vi "Galvo Parameters - FGV.vi"(7 "Actions":T19=enum."Clear", 8 "Error In":errorcluster, 10 "Galvo parameters in":T1={"System Parameters"={"Optical Parameters"={"Obj. Focal Length [mm]"=45.0, "Scan Lens EFL[mm]"=59.5, "Tube Lens EFL[mm]"=205.0, "Galvo V Range (+/-)"=10.0, "Galvo Max Half Angle [Deg]"=19.0, "Max Galvo Range[%]"=0.0}, "Vibratome"={"Z Bottom [mm]"=0.0, "Pre Cut Dwell [s]"=0.0, "Blade Frequency [RPM]"=0, "Slice Speed [mm/s]"=0.0, "Post Cut Dwell [s]"=0.0, "Ramp Time [s]"=0.0, "Start X [mm]"=0.0, "Start Y [mm]"=0.0, "Slice Length [mm]"=0.0, "Slice Axis"=enum."Y Axis", "Controller VISA Ref"="COM4"}, "Table Stages"={"X Stage"={"Position"=0.0, "Is.Enabled?"=FALSE, "Is.Connected?"=FALSE, "Device SN"="45876539", "AccelerationMaximum"=0.0, "VelocityMaximum"=0.0, "Acceleration"=0.0, "Velocity"=0.0, "waitTimeout (ms)"=0, "Model"=enum."None", "Is.Homed?"=FALSE}, "Y Stage"={"Position"=0.0, "Is.Enabled?"=FALSE, "Is.Connected?"=FALSE, "Device SN"="45876539", "AccelerationMaximum"=0.0, "VelocityMaximum"=0.0, "Acceleration"=0.0, "Velocity"=0.0, "waitTimeout (ms)"=0, "Model"=enum."None", "Is.Homed?"=FALSE}, "Z Stage"={"Position"=0.0, "Is.Enabled?"=FALSE, "Is.Connected?"=FALSE, "Device SN"="45876539", "AccelerationMaximum"=0.0, "VelocityMaximum"=0.0, "Acceleration"=0.0, "Velocity"=0.0, "waitTimeout (ms)"=0, "Model"=enum."None", "Is.Homed?"=FALSE}}, "Imaging Parameter"={"Raster Scan Direction"=enum."Uni Directional", "Pixel Dwell Time [Clock Cycles]"=1, "Flyback Time [Clock Cycles]"=200, "XY Center [um]"={"X"=1.0, "Y"=1.0}, "Pixel Step Size [um]"=2.5, "XY Image Size"=enum."2048 x 2048", "Custom"=FALSE, "Custom Size"={"X"=10, "Y"=10}, "Line Averages"=1}, "Galvo HW Parameters"={"Analog Out Channel"="GalvoCtrl/ao0,GalvoCtrl/ao1", "Min Voltage"=-10.0, "Max Voltage"=10.0, "Pixel Clock Source"="/GalvoCtrl/PFI0", "Sample Rate"=1000.0, "Line Clock Out Ch"="GalvoCtrl/port0/line0"}, "Alazar parameters"={"Trigger Settings"={"General Trigger Settings"={"Trigger Operation"=0, "Coupling ID"=2, "Range ID"=2, "Delay"=0, "Timeout Ticks"=0, "Mode"=1, "Parameter"=1}, "Trigger Engine 1"={"Trigger Engine"=0, "Source"=2, "Slope"=1, "Level"=140}, "Trigger Engine 2"={"Trigger Engine"=1, "Source"=3, "Slope"=1, "Level"=140}}, "Capture Clock"={"Sample Rate"=100, "Decimation"=0, "Source"=2, "Edge"=0}, "Device ID"={"System ID"=1, "Board ID"=1}, "Ch A Input Control"={"Channel"=1, "Coupling"=2, "Range"=10, "Impedance"=2}, "Ch B Input Control"={"Channel"=2, "Coupling"=2, "Range"=10, "Impedance"=2}, "Acq Settings"={"Window Type"=1, "Record Length"=1440, "Footer"=0, "Output Format"=10, "Offset"=0, "Records Per Buffer"=2048, "Samples per record"=2048, "Records Count (Records/Acq)"=2147483647}, "Cluster"={"FFT value magnification"=1000.0, "max queue size (-1, unlimited)"=-1, "File Type"=enum."Tiff", "file path"=path "C:/Users/BoasLab/Documents/Data/Alazar data/B-line/data/test.tif", "#A-lines to save"=2048, "#Z pixels to save"=2048, "ImageDescription"="", "Convert to U16?"=FALSE}}}} {"System Parameters"."Alazar parameters"."Cluster"."FFT value magnification" min=0.0 max=10000.0 step=0.001 format="%.4f"; "System Parameters"."Alazar parameters"."Acq Settings"."Window Type" items=["DSP_WINDOW_NONE", "DSP_WINDOW_HANNING", "DSP_WINDOW_HAMMING", "DSP_WINDOW_BLACKMAN", "DSP_WINDOW_BLACKMAN_HARRIS", "DSP_WINDOW_BARTLETT"]; "System Parameters"."Alazar parameters"."Acq Settings"."Footer" items=["FOOTER_NONE", "FOOTER_NPT"]; "System Parameters"."Alazar parameters"."Acq Settings"."Output Format" items=["FLOAT_AMP2"=10, "FLOAT_LOG"=11]; "System Parameters"."Alazar parameters"."Ch B Input Control"."Channel" items=["A"=1, "B"=2, "C"=4, "D"=8]; "System Parameters"."Alazar parameters"."Ch B Input Control"."Coupling" items=["AC"=1, "DC"=2]; "System Parameters"."Alazar parameters"."Ch B Input Control"."Range" items=["20 mV"=1, "40 mV"=2, "50 mV"=3, "80 mV"=4, "100 mV"=5, "200 mV"=6, "400 mV"=7, "500 mV"=8, "800 mV"=9, "1 V"=10, "1.25 V"=33, "2 V"=11, "4 V"=12, "5 V"=13, "8 V"=14, "10 V"=15, "20 V"=16]; "System Parameters"."Alazar parameters"."Ch B Input Control"."Impedance" items=["1 MOhm"=1, "50 Ohm"=2, ""=0]; "System Parameters"."Alazar parameters"."Ch A Input Control"."Channel" items=["A"=1, "B"=2, "C"=4, "D"=8]; "System Parameters"."Alazar parameters"."Ch A Input Control"."Coupling" items=["AC"=1, "DC"=2]; "System Parameters"."Alazar parameters"."Ch A Input Control"."Range" items=["20 mV"=1, "40 mV"=2, "50 mV"=3, "80 mV"=4, "100 mV"=5, "200 mV"=6, "400 mV"=7, "500 mV"=8, "800 mV"=9, "1 V"=10, "1.25 V"=33, "2 V"=11, "4 V"=12, "5 V"=13, "8 V"=14, "10 V"=15, "20 V"=16]; "System Parameters"."Alazar parameters"."Ch A Input Control"."Impedance" items=["1 MOhm"=1, "50 Ohm"=2, ""=0]; "System Parameters"."Alazar parameters"."Capture Clock"."Edge" items=["Rising", "Falling"]; "System Parameters"."Alazar parameters"."Capture Clock"."Source" items=["Internal"=1, "Fast External"=2, "Medium External"=3, "Slow External"=4, "External AC"=5, "External DC"=6, "External 10MHz"=7]; "System Parameters"."Alazar parameters"."Trigger Settings"."General Trigger Settings"."Trigger Operation" items=["J", "K", "J OR K", "J AND K", "J XOR K", "J AND NOT K", "NOT J AND K"]; "System Parameters"."Alazar parameters"."Trigger Settings"."General Trigger Settings"."Coupling ID" items=["AC"=1, "DC"=2]; "System Parameters"."Alazar parameters"."Trigger Settings"."General Trigger Settings"."Range ID" items=["5 V", "1 V", "TTL"]; "System Parameters"."Alazar parameters"."Trigger Settings"."Trigger Engine 1"."Trigger Engine" items=["J", "K"]; "System Parameters"."Alazar parameters"."Trigger Settings"."Trigger Engine 1"."Source" items=["A", "B", "External", "Disable", "C", "D"]; "System Parameters"."Alazar parameters"."Trigger Settings"."Trigger Engine 1"."Slope" items=["Positive"=1, "Negative"=2]; "System Parameters"."Alazar parameters"."Trigger Settings"."Trigger Engine 2"."Trigger Engine" items=["J", "K"]; "System Parameters"."Alazar parameters"."Trigger Settings"."Trigger Engine 2"."Source" items=["A", "B", "External", "Disable", "C", "D"]; "System Parameters"."Alazar parameters"."Trigger Settings"."Trigger Engine 2"."Slope" items=["Positive"=1, "Negative"=2]; "System Parameters"."Imaging Parameter"."Line Averages" min=1 max=30 step=1; "System Parameters"."Imaging Parameter"."Flyback Time [Clock Cycles]" max=10 step=1; "System Parameters"."Imaging Parameter"."Pixel Step Size [um]" min=0.0 max=10.0 step=0.01; "System Parameters"."Imaging Parameter"."Custom Size"."Y" min=1 max=30 step=1; "System Parameters"."Imaging Parameter"."Custom Size"."X" min=1 max=30 step=1; "System Parameters"."Imaging Parameter"."XY Center [um]"."Y" min=1.0 max=30.0 step=1.0; "System Parameters"."Imaging Parameter"."XY Center [um]"."X" min=1.0 max=30.0 step=1.0; "System Parameters"."Imaging Parameter"."Pixel Dwell Time [Clock Cycles]" max=10 step=1}) -> (0 "Error Out":errorcluster, 2 "Galvo parameters out":T1={"System Parameters"={"Optical Parameters"={"Obj. Focal Length [mm]"=45.0, "Scan Lens EFL[mm]"=59.5, "Tube Lens EFL[mm]"=205.0, "Galvo V Range (+/-)"=10.0, "Galvo Max Half Angle [Deg]"=19.0, "Max Galvo Range[%]"=0.0}, "Vibratome"={"Z Bottom [mm]"=0.0, "Pre Cut Dwell [s]"=0.0, "Blade Frequency [RPM]"=0, "Slice Speed [mm/s]"=0.0, "Post Cut Dwell [s]"=0.0, "Ramp Time [s]"=0.0, "Start X [mm]"=0.0, "Start Y [mm]"=0.0, "Slice Length [mm]"=0.0, "Slice Axis"=enum."Y Axis", "Controller VISA Ref"="COM4"}, "Table Stages"={"X Stage"={"Position"=0.0, "Is.Enabled?"=FALSE, "Is.Connected?"=FALSE, "Device SN"="45876539", "AccelerationMaximum"=0.0, "VelocityMaximum"=0.0, "Acceleration"=0.0, "Velocity"=0.0, "waitTimeout (ms)"=0, "Model"=enum."None", "Is.Homed?"=FALSE}, "Y Stage"={"Position"=0.0, "Is.Enabled?"=FALSE, "Is.Connected?"=FALSE, "Device SN"="45876539", "AccelerationMaximum"=0.0, "VelocityMaximum"=0.0, "Acceleration"=0.0, "Velocity"=0.0, "waitTimeout (ms)"=0, "Model"=enum."None", "Is.Homed?"=FALSE}, "Z Stage"={"Position"=0.0, "Is.Enabled?"=FALSE, "Is.Connected?"=FALSE, "Device SN"="45876539", "AccelerationMaximum"=0.0, "VelocityMaximum"=0.0, "Acceleration"=0.0, "Velocity"=0.0, "waitTimeout (ms)"=0, "Model"=enum."None", "Is.Homed?"=FALSE}}, "Imaging Parameter"={"Raster Scan Direction"=enum."Uni Directional", "Pixel Dwell Time [Clock Cycles]"=1, "Flyback Time [Clock Cycles]"=200, "XY Center [um]"={"X"=1.0, "Y"=1.0}, "Pixel Step Size [um]"=2.5, "XY Image Size"=enum."2048 x 2048", "Custom"=FALSE, "Custom Size"={"X"=10, "Y"=10}, "Line Averages"=1}, "Galvo HW Parameters"={"Analog Out Channel"="GalvoCtrl/ao0,GalvoCtrl/ao1", "Min Voltage"=-10.0, "Max Voltage"=10.0, "Pixel Clock Source"="/GalvoCtrl/PFI0", "Sample Rate"=1000.0, "Line Clock Out Ch"="GalvoCtrl/port0/line0"}, "Alazar parameters"={"Trigger Settings"={"General Trigger Settings"={"Trigger Operation"=0, "Coupling ID"=2, "Range ID"=2, "Delay"=0, "Timeout Ticks"=0, "Mode"=1, "Parameter"=1}, "Trigger Engine 1"={"Trigger Engine"=0, "Source"=2, "Slope"=1, "Level"=140}, "Trigger Engine 2"={"Trigger Engine"=1, "Source"=3, "Slope"=1, "Level"=140}}, "Capture Clock"={"Sample Rate"=100, "Decimation"=0, "Source"=2, "Edge"=0}, "Device ID"={"System ID"=1, "Board ID"=1}, "Ch A Input Control"={"Channel"=1, "Coupling"=2, "Range"=10, "Impedance"=2}, "Ch B Input Control"={"Channel"=2, "Coupling"=2, "Range"=10, "Impedance"=2}, "Acq Settings"={"Window Type"=1, "Record Length"=1440, "Footer"=0, "Output Format"=10, "Offset"=0, "Records Per Buffer"=2048, "Samples per record"=2048, "Records Count (Records/Acq)"=2147483647}, "Cluster"={"FFT value magnification"=1000.0, "max queue size (-1, unlimited)"=-1, "File Type"=enum."Tiff", "file path"=path "C:/Users/BoasLab/Documents/Data/Alazar data/B-line/data/test.tif", "#A-lines to save"=2048, "#Z pixels to save"=2048, "ImageDescription"="", "Convert to U16?"=FALSE}}}} {"System Parameters"."Alazar parameters"."Cluster"."FFT value magnification" min=0.0 max=10000.0 step=0.001 format="%.4f"; "System Parameters"."Alazar parameters"."Acq Settings"."Window Type" items=["DSP_WINDOW_NONE", "DSP_WINDOW_HANNING", "DSP_WINDOW_HAMMING", "DSP_WINDOW_BLACKMAN", "DSP_WINDOW_BLACKMAN_HARRIS", "DSP_WINDOW_BARTLETT"]; "System Parameters"."Alazar parameters"."Acq Settings"."Footer" items=["FOOTER_NONE", "FOOTER_NPT"]; "System Parameters"."Alazar parameters"."Acq Settings"."Output Format" items=["FLOAT_AMP2"=10, "FLOAT_LOG"=11]; "System Parameters"."Alazar parameters"."Ch B Input Control"."Channel" items=["A"=1, "B"=2, "C"=4, "D"=8]; "System Parameters"."Alazar parameters"."Ch B Input Control"."Coupling" items=["AC"=1, "DC"=2]; "System Parameters"."Alazar parameters"."Ch B Input Control"."Range" items=["20 mV"=1, "40 mV"=2, "50 mV"=3, "80 mV"=4, "100 mV"=5, "200 mV"=6, "400 mV"=7, "500 mV"=8, "800 mV"=9, "1 V"=10, "1.25 V"=33, "2 V"=11, "4 V"=12, "5 V"=13, "8 V"=14, "10 V"=15, "20 V"=16]; "System Parameters"."Alazar parameters"."Ch B Input Control"."Impedance" items=["1 MOhm"=1, "50 Ohm"=2, ""=0]; "System Parameters"."Alazar parameters"."Ch A Input Control"."Channel" items=["A"=1, "B"=2, "C"=4, "D"=8]; "System Parameters"."Alazar parameters"."Ch A Input Control"."Coupling" items=["AC"=1, "DC"=2]; "System Parameters"."Alazar parameters"."Ch A Input Control"."Range" items=["20 mV"=1, "40 mV"=2, "50 mV"=3, "80 mV"=4, "100 mV"=5, "200 mV"=6, "400 mV"=7, "500 mV"=8, "800 mV"=9, "1 V"=10, "1.25 V"=33, "2 V"=11, "4 V"=12, "5 V"=13, "8 V"=14, "10 V"=15, "20 V"=16]; "System Parameters"."Alazar parameters"."Ch A Input Control"."Impedance" items=["1 MOhm"=1, "50 Ohm"=2, ""=0]; "System Parameters"."Alazar parameters"."Capture Clock"."Edge" items=["Rising", "Falling"]; "System Parameters"."Alazar parameters"."Capture Clock"."Source" items=["Internal"=1, "Fast External"=2, "Medium External"=3, "Slow External"=4, "External AC"=5, "External DC"=6, "External 10MHz"=7]; "System Parameters"."Alazar parameters"."Trigger Settings"."General Trigger Settings"."Trigger Operation" items=["J", "K", "J OR K", "J AND K", "J XOR K", "J AND NOT K", "NOT J AND K"]; "System Parameters"."Alazar parameters"."Trigger Settings"."General Trigger Settings"."Coupling ID" items=["AC"=1, "DC"=2]; "System Parameters"."Alazar parameters"."Trigger Settings"."General Trigger Settings"."Range ID" items=["5 V", "1 V", "TTL"]; "System Parameters"."Alazar parameters"."Trigger Settings"."Trigger Engine 1"."Trigger Engine" items=["J", "K"]; "System Parameters"."Alazar parameters"."Trigger Settings"."Trigger Engine 1"."Source" items=["A", "B", "External", "Disable", "C", "D"]; "System Parameters"."Alazar parameters"."Trigger Settings"."Trigger Engine 1"."Slope" items=["Positive"=1, "Negative"=2]; "System Parameters"."Alazar parameters"."Trigger Settings"."Trigger Engine 2"."Trigger Engine" items=["J", "K"]; "System Parameters"."Alazar parameters"."Trigger Settings"."Trigger Engine 2"."Source" items=["A", "B", "External", "Disable", "C", "D"]; "System Parameters"."Alazar parameters"."Trigger Settings"."Trigger Engine 2"."Slope" items=["Positive"=1, "Negative"=2]; "System Parameters"."Imaging Parameter"."Line Averages" min=1 max=30 step=1; "System Parameters"."Imaging Parameter"."Flyback Time [Clock Cycles]" max=10 step=1; "System Parameters"."Imaging Parameter"."Pixel Step Size [um]" min=0.0 max=10.0 step=0.01; "System Parameters"."Imaging Parameter"."Custom Size"."Y" min=1 max=30 step=1; "System Parameters"."Imaging Parameter"."Custom Size"."X" min=1 max=30 step=1; "System Parameters"."Imaging Parameter"."XY Center [um]"."Y" min=1.0 max=30.0 step=1.0; "System Parameters"."Imaging Parameter"."XY Center [um]"."X" min=1.0 max=30.0 step=1.0; "System Parameters"."Imaging Parameter"."Pixel Dwell Time [Clock Cycles]" max=10 step=1})   [LabVIEW 2018]
uses:
  Controls/FGV Actions.ctl
  type defines/Galvo parameters.ctl
  Controls/System Parameters.ctl
  Controls/Optical Parameters.ctl
  Controls/Vibratome Parameters.ctl
  Controls/Translation Stage Parameters.ctl
  Hardware Mfg/Thorlabs Translation Stages/Controls/Translation Stage Cluster.ctl
  Controls/Translation Stage Types.ctl
  Controls/Imaging Parameters.ctl
  Controls/Scan Direction.ctl
  type defines/Alazar parameters.ctl
  Hardware Mfg/AlazarTech SDK/Controls/General Trigger Settings.ctl
  Hardware Mfg/AlazarTech SDK/Controls/Trigger Engine Controls.ctl
  Hardware Mfg/AlazarTech SDK/Controls/Clock Controls.ctl
  Hardware Mfg/AlazarTech SDK/Controls/Alazar Device ID.ctl
  Hardware Mfg/AlazarTech SDK/Controls/Channel Input Controls.ctl
  Hardware Mfg/AlazarTech SDK/Controls/Alazar Acquisition Settings.ctl
  Controls/Control cluster.ctl
  type defines/file type.ctl
panel:
  # "X"
  # "X"
  # "X"
  # "X"
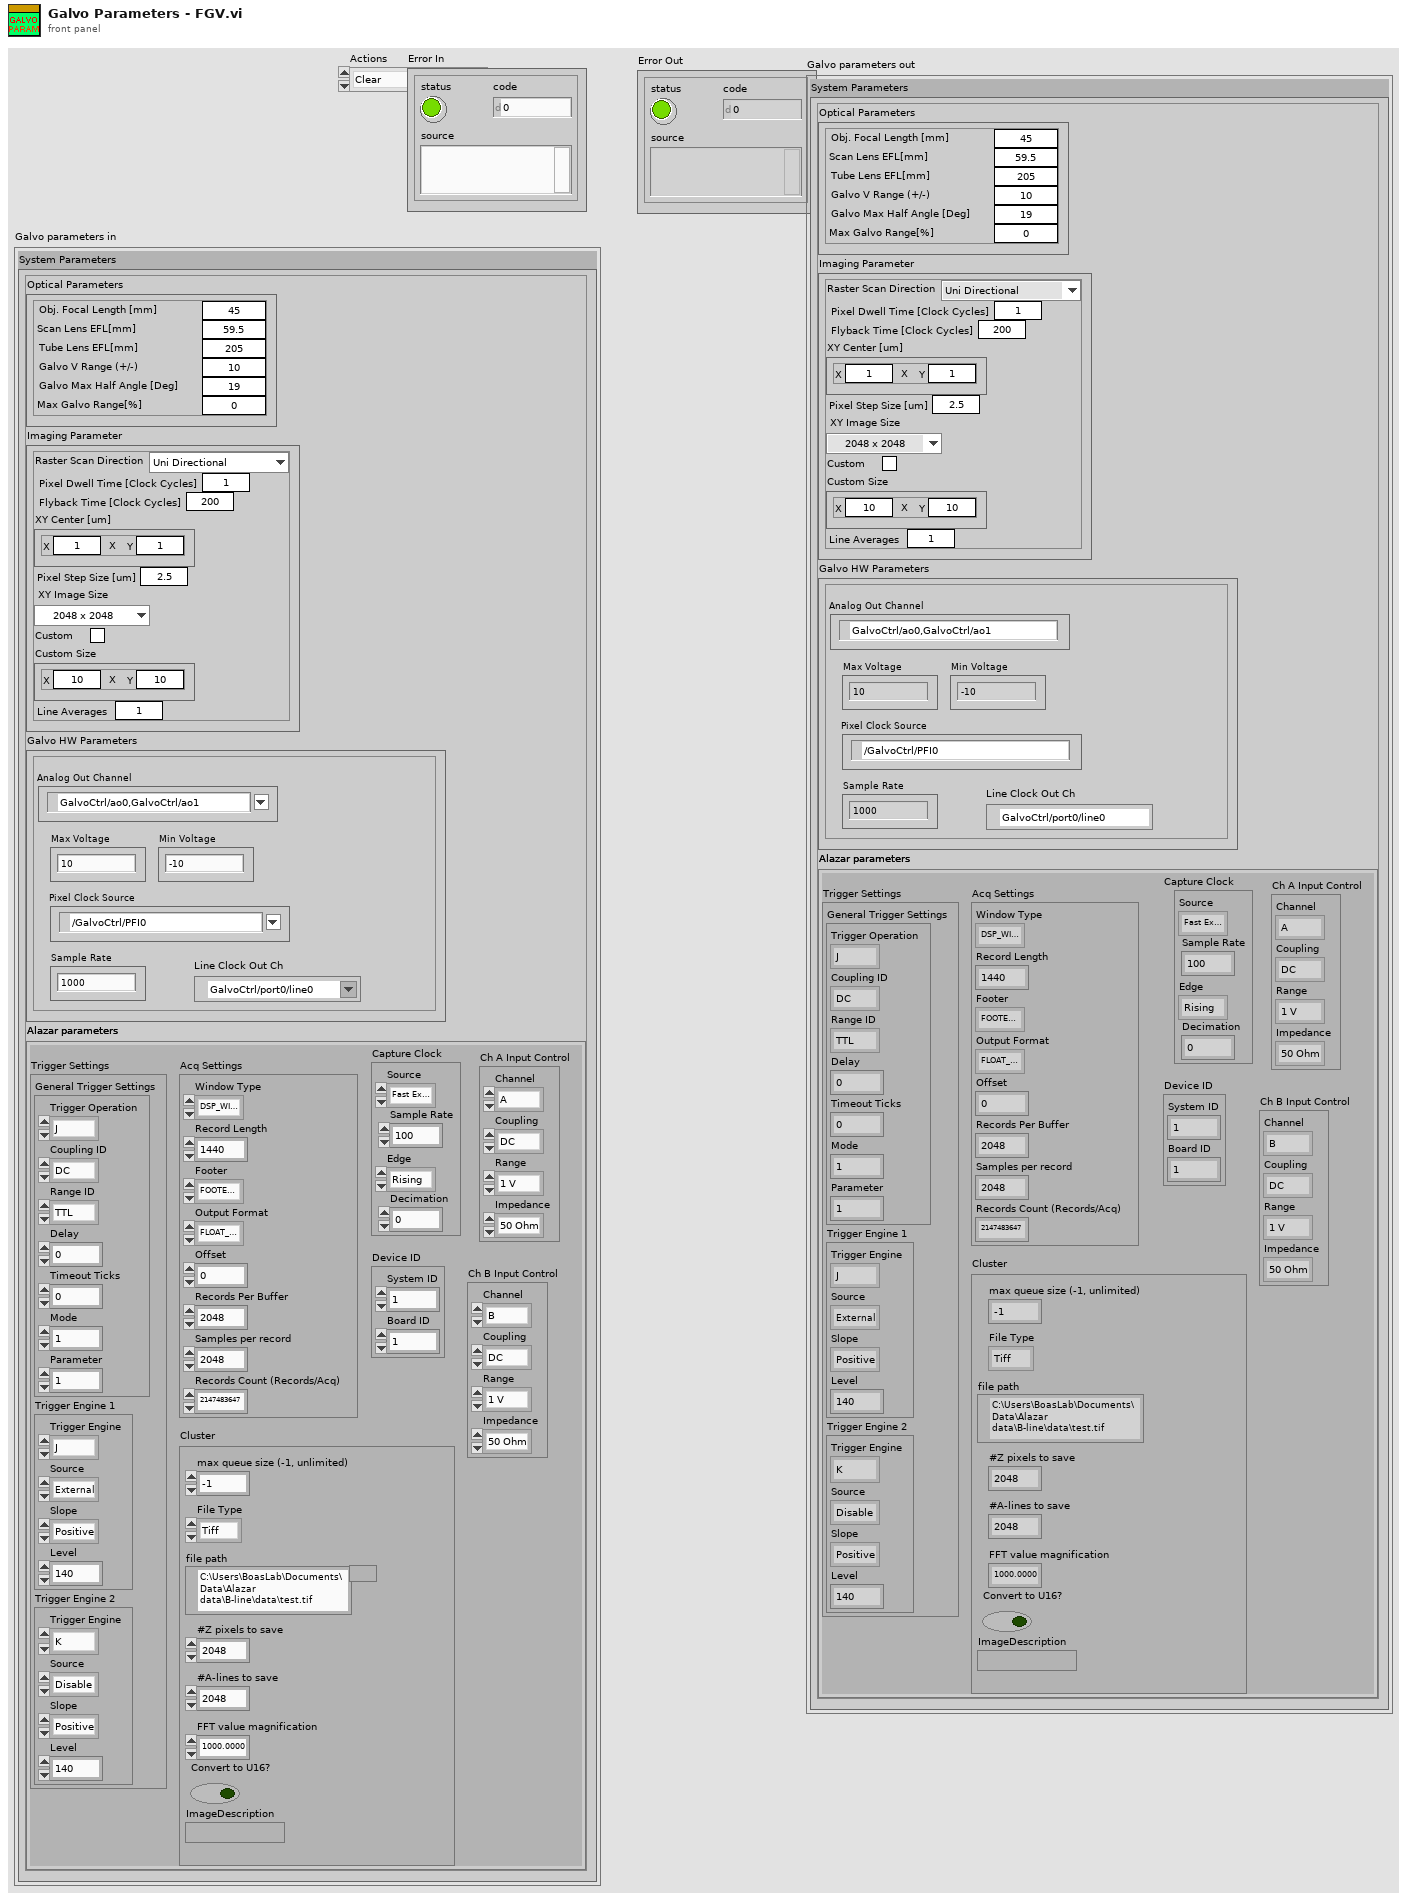
[diagram p1: front panel]
types:
  T1 = typedef "Galvo parameters.ctl" = cluster{"System Parameters":T2}
  T2 = typedef "System Parameters.ctl" = cluster{"Optical Parameters":T3, "Vibratome":T4, "Table Stages":T5, "Imaging Parameter":T8, "Galvo HW Parameters":cluster{"Analog Out Channel":tag, "Min Voltage":dbl, "Max Voltage":dbl, "Pixel Clock Source":tag, "Sample Rate":dbl, "Line Clock Out Ch":tag}, "Alazar parameters":T10}
  T3 = typedef "Optical Parameters.ctl" = cluster{"Obj. Focal Length [mm]":dbl, "Scan Lens EFL[mm]":dbl, "Tube Lens EFL[mm]":dbl, "Galvo V Range (+/-)":dbl, "Galvo Max Half Angle [Deg]":dbl, "Max Galvo Range[%]":dbl}
  T4 = typedef "Vibratome Parameters.ctl" = cluster{"Z Bottom [mm]":dbl, "Pre Cut Dwell [s]":dbl, "Blade Frequency [RPM]":u16, "Slice Speed [mm/s]":dbl, "Post Cut Dwell [s]":dbl, "Ramp Time [s]":dbl, "Start X [mm]":dbl, "Start Y [mm]":dbl, "Slice Length [mm]":dbl, "Slice Axis":enum16{"X Axis", "Y Axis", "Z Axis"}, "Controller VISA Ref":refnum<visa-resource-name>}
  T5 = typedef "Translation Stage Parameters.ctl" = cluster{"X Stage":T6, "Y Stage":T6, "Z Stage":T6}
  T6 = typedef "Translation Stage Cluster.ctl" = cluster{"Position":dbl, "Is.Enabled?":bool, "Is.Connected?":bool, "Device SN":string, "AccelerationMaximum":dbl, "VelocityMaximum":dbl, "Acceleration":dbl, "Velocity":dbl, "waitTimeout (ms)":i32, "Model":T7, "Is.Homed?":bool}
  T7 = typedef "Translation Stage Types.ctl" = enum16{"None", "Thorlabs LTS", "Thorlabs MLJ"}
  T8 = typedef "Imaging Parameters.ctl" = cluster{"Raster Scan Direction":T9, "Pixel Dwell Time [Clock Cycles]":u16, "Flyback Time [Clock Cycles]":u16, "XY Center [um]":cluster{"X":dbl, "Y":dbl}, "Pixel Step Size [um]":dbl, "XY Image Size":enum16{"32 x 32", "64 x 64", "128 x 128", "256 x 256", "512 x 512", "1024 x 1024", "2048 x 2048"}, "Custom":bool, "Custom Size":cluster{"X":u16, "Y":u16}, "Line Averages":u8}
  T9 = typedef "Scan Direction.ctl" = enum16{"Uni Directional", "Bi Directional", "None"}
  T10 = typedef "Alazar parameters.ctl" = cluster{"Trigger Settings":cluster{"General Trigger Settings":T11, "Trigger Engine 1":T12, "Trigger Engine 2":T12}, "Capture Clock":T13, "Device ID":T14, "Ch A Input Control":T15, "Ch B Input Control":T15, "Acq Settings":T16, "Cluster":T17}
  T11 = typedef "General Trigger Settings.ctl" = cluster{"Trigger Operation":u32, "Coupling ID":u32, "Range ID":u32, "Delay":u32, "Timeout Ticks":u32, "Mode":u32, "Parameter":u32}
  T12 = typedef "Trigger Engine Controls.ctl" = cluster{"Trigger Engine":u32, "Source":u32, "Slope":u32, "Level":u32}
  T13 = typedef "Clock Controls.ctl" = cluster{"Sample Rate":u32, "Decimation":u32, "Source":u32, "Edge":u32}
  T14 = typedef "Alazar Device ID.ctl" = cluster{"System ID":u32, "Board ID":u32}
  T15 = typedef "Channel Input Controls.ctl" = cluster{"Channel":u8, "Coupling":u32, "Range":u32, "Impedance":u32}
  T16 = typedef "Alazar Acquisition Settings.ctl" = cluster{"Window Type":u32, "Record Length":u32, "Footer":u32, "Output Format":u32, "Offset":u32, "Records Per Buffer":u32, "Samples per record":u32, "Records Count (Records/Acq)":u32}
  T17 = typedef "Control cluster.ctl" = cluster{"FFT value magnification":dbl, "max queue size (-1, unlimited)":i32, "File Type":T18, "file path":path, "#A-lines to save":u32, "#Z pixels to save":u32, "ImageDescription":string, "Convert to U16?":bool}
  T18 = typedef "file type.ctl" = enum16{"text", "Tiff", "binary"}
  T19 = typedef "FGV Actions.ctl" = enum16{"Init", "Set", "Get", "Clear"}
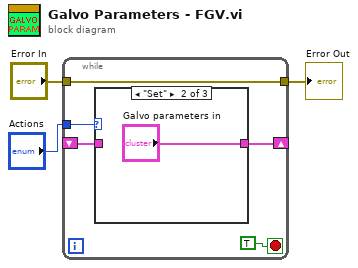
[diagram p0: block diagram]
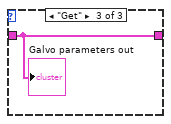
[diagram p3: hidden frame]
diagram:
  n1 = while {
    tunnel: "Actions" -> [w6]
    shift-right: [w7] -> _
    shift-left: _ -> [w5]
    tunnel: "Error In" -> [w4]
    tunnel: [w4] -> w1
    stop <- TRUE stop-if-true
    n2 = case shown="\"Set\"" w6 {
      tunnel: [_ "Galvo parameters in" w10] -> w7
      tunnel: w5 -> [_ _ w10]
      frame "Init", Default {
      }
      frame "Set" {
      }
      frame "Get" {
        "Galvo parameters out" <- w10
      }
    }
  }
  "Error Out" <- w1
